vi "20TVTI_Merge_Cluster.vi"(1 "VTI Control":T3, 2 "VTI Status":T2={"Temperatur (K)"=70.6986, "Heater (%)"=0.0017142857142857142, "NV (%)"=0.0, "Heater Manual"=TRUE, "NV Manual"=TRUE, "Pressure"=1.0208606, "Dewar Pressure"=1.0500276, "Valid?"=FALSE, "Dewar Heater Manual"=FALSE, "Heater (%) Display"=0.0, "NV (%) Display"=0.0, "Dewar Heater (%)"=18.434412358753207, "D-Heater (%) Display"=18.434412358753207} {"Heater (%)" scale=0.0..100.0; "NV (%)" scale=0.0..100.0; "Dewar Heater (%)" scale=0.0..100.0}) -> (0 "VTI Cluster":T1={"Temperatur (K)"=70.6986, "Setpoint (K)"=0.0, "Rate (K/min)"=3.4572, "Heater (%)"=0.0017142857142857142, "NV (%)"=0.0, "Heater Manual"=TRUE, "NV Manual"=TRUE, "Go to Set"=FALSE, "Pressure"=1.0208606, "Heater SP"=0.0, "Valid?"=FALSE, "Set Heater SP"=FALSE, "Set NV SP"=FALSE, "Heater (%) Display"=0.0, "NV (%) Display"=0.0, "NV Setpoint"=0.0, "Change Heater Status"=FALSE, "Change NV Status"=FALSE, "Change Sweep Type"=FALSE} {"NV (%) Display" format="%4_5f"; "Heater (%) Display" format="%4_5f"; "Heater SP" format="%#4_5f"; "Pressure" format="%#4_5f"; "NV (%)" scale=0.0..100.0; "Heater (%)" scale=0.0..100.0; "Rate (K/min)" format="%#4_5f"; "Setpoint (K)" format="%6_5f"})   [LabVIEW 2018]
uses:
  Gustav/20TVTI_Control.ctl
  Gustav/20TVTI_Status.ctl
  Gustav/20TVTI_Cluster.ctl
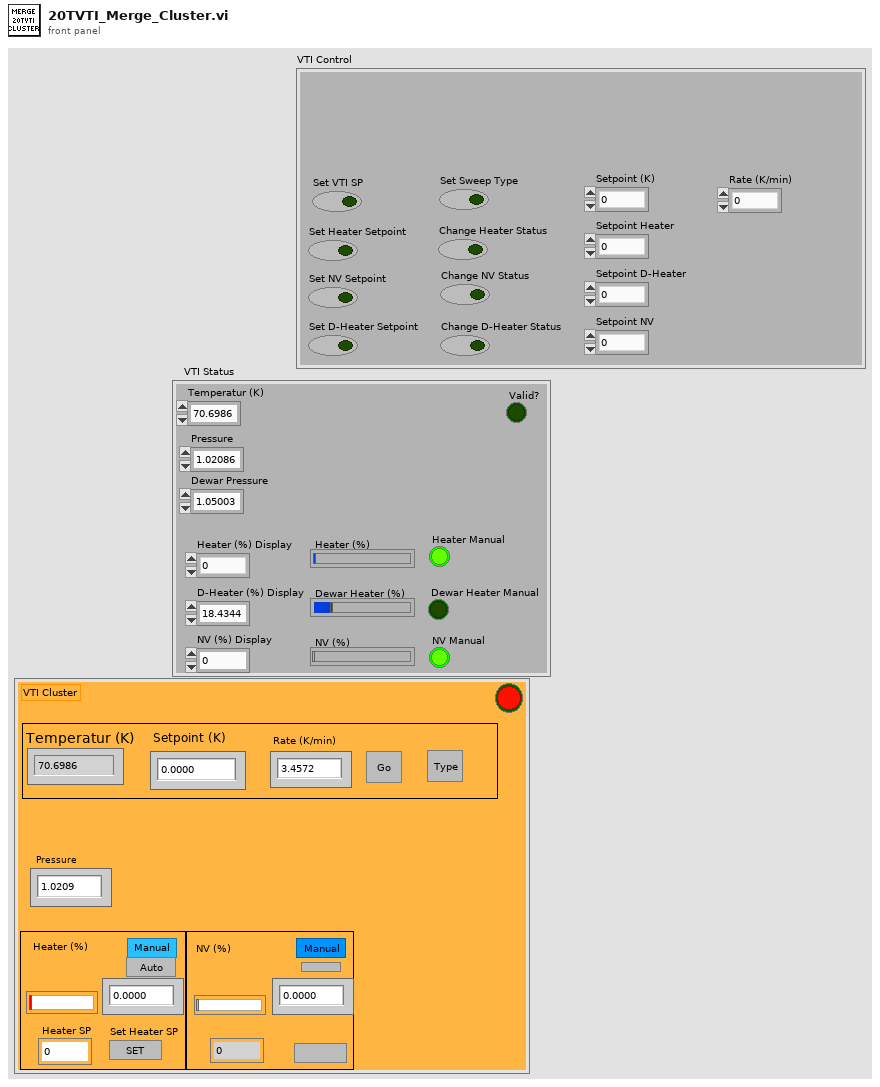
[diagram p1: front panel]
types:
  T1 = typedef "20TVTI_Cluster.ctl" = cluster{"Temperatur (K)":dbl, "Setpoint (K)":dbl, "Rate (K/min)":dbl, "Heater (%)":dbl, "NV (%)":dbl, "Heater Manual":bool, "NV Manual":bool, "Go to Set":bool, "Pressure":dbl, "Heater SP":dbl, "Valid?":bool, "Set Heater SP":bool, "Set NV SP":bool, "Heater (%) Display":dbl, "NV (%) Display":dbl, "NV Setpoint":dbl, "Change Heater Status":bool, "Change NV Status":bool, "Change Sweep Type":bool}
  T2 = typedef "20TVTI_Status.ctl" = cluster{"Temperatur (K)":dbl, "Heater (%)":dbl, "NV (%)":dbl, "Heater Manual":bool, "NV Manual":bool, "Pressure":dbl, "Dewar Pressure":dbl, "Valid?":bool, "Dewar Heater Manual":bool, "Heater (%) Display":dbl, "NV (%) Display":dbl, "Dewar Heater (%)":dbl, "D-Heater (%) Display":dbl}
  T3 = typedef "20TVTI_Control.ctl" = cluster{"Set VTI SP":bool, "Change NV Status":bool, "Set NV Setpoint":bool, "Change Heater Status":bool, "Set D-Heater Setpoint":bool, "Set Heater Setpoint":bool, "Change D-Heater Status":bool, "Set Sweep Type":bool, "Setpoint (K)":dbl, "Rate (K/min)":dbl, "Setpoint Heater":dbl, "Setpoint D-Heater":dbl, "Setpoint NV":dbl}
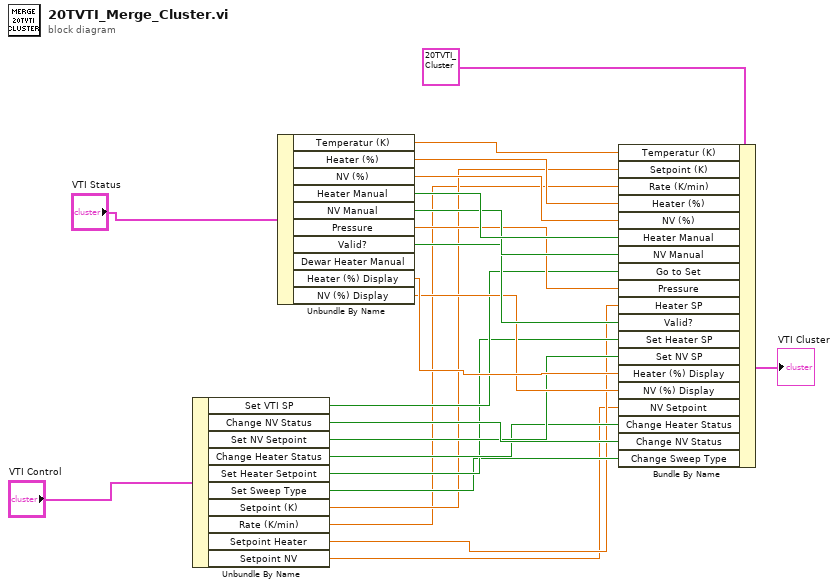
[diagram p0: block diagram]
diagram:
  n1 = Unbundle By Name("VTI Control") -> ("Set VTI SP"=w11:bool, "Change NV Status"=w10:bool, "Set NV Setpoint"=w9:bool, "Change Heater Status"=w8:bool, "Set Heater Setpoint"=w7:bool, "Set Sweep Type"=w6:bool, "Setpoint (K)"=w5:dbl, "Rate (K/min)"=w4:dbl, "Setpoint Heater"=w3:dbl, "Setpoint NV"=w2:dbl)
  n2 = Unbundle By Name("VTI Status") -> ("Temperatur (K)"=w20:dbl, "Heater (%)"=w19:dbl, "NV (%)"=w18:dbl, "Heater Manual"=w17:bool, "NV Manual"=w16:bool, "Pressure"=w15:dbl, "Valid?"=w14:bool, "Heater (%) Display"=w13:dbl, "NV (%) Display"=w12:dbl)  [unwired: 1 out]
  n3 = Bundle By Name(cluster=T1 {"Temperatur (K)"=70.6986, "Setpoint (K)"=0.0, "Rate (K/min)"=3.4572, "Heater (%)"=0.0017142857142857142, "NV (%)"=0.0, "Heater Manual"=TRUE, "NV Manual"=TRUE, "Go to Set"=FALSE, "Pressure"=1.0208606, "Heater SP"=0.0, "Valid?"=FALSE, "Set Heater SP"=FALSE, "Set NV SP"=FALSE, "Heater (%) Display"=0.0, "NV (%) Display"=0.0, "NV Setpoint"=0.0, "Change Heater Status"=FALSE, "Change NV Status"=FALSE, "Change Sweep Type"=FALSE} ("VTI Cluster 2"), "Temperatur (K)"=w20, "Setpoint (K)"=w5, "Rate (K/min)"=w4, "Heater (%)"=w19, "NV (%)"=w18, "Heater Manual"=w17, "NV Manual"=w16, "Go to Set"=w11, "Pressure"=w15, "Heater SP"=w3, "Valid?"=w14, "Set Heater SP"=w7, "Set NV SP"=w9, "Heater (%) Display"=w13, "NV (%) Display"=w12, "NV Setpoint"=w2, "Change Heater Status"=w8, "Change NV Status"=w10, "Change Sweep Type"=w6) -> (→"VTI Cluster":T1)
